vi "Set Scroll Bar State.vi"(8 "Error In":errorcluster, 10 "Scrollbar Visibility (Always On)":T1(ring), 11 "Pane Ref In":refnum<vi>) -> (0 "Error Out":errorcluster, 3 "Pane Ref Out":refnum<vi>)   [LabVIEW 2014]
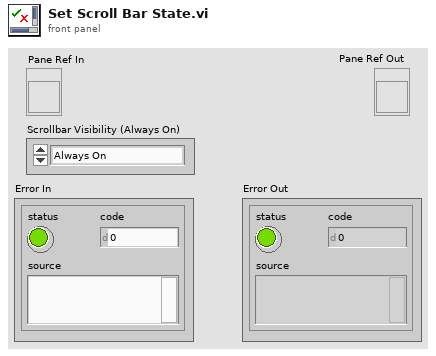
[diagram p1: front panel]
types:
  T1 = enum16{"Always On", "Always Off", "Off While Running"}
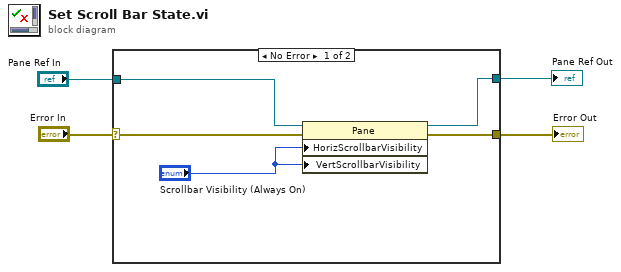
[diagram p0: block diagram]
diagram:
  n1 = case shown="No Error" "Error In" {
    selector: "Error In" -> [w8 w11]
    tunnel: [w7 w11] -> w3
    tunnel: "Pane Ref In" -> [w9 w10]
    tunnel: [w6 w10] -> w1
    frame No Error {
      n2 = property class="Pane"(reference=w9, error in=w8, "HorizScrollbarVisibility"="Scrollbar Visibility (Always On)", "VertScrollbarVisibility"="Scrollbar Visibility (Always On)") -> (reference out=w6:refnum<vi>, error out=w7:errorcluster)
    }
    frame Error {
    }
  }
  "Error Out" <- w3
  "Pane Ref Out" <- w1
